vi "Sequence Read.vi"(8 "error in (no error)":errorcluster, 11 "CAP-USB-1 in":refnum<class "CAP-USB-1.lvclass">) -> (0 "error out":errorcluster, 1 "Control Data":T3, 2 "Acquisition Data":T1, 3 "CAP-USB-1 out":refnum<class "CAP-USB-1.lvclass">)   [LabVIEW 2014, in "CAP-USB-1.lvlib" / "CAP-USB-1.lvclass"]
doc: "Realiza la lectura de los valores enviados por el dispositivo en modo sequence"
uses:
  CAP-USB-1.lvclass
  DriverMasterSync/build/DriverMasterSync.lvlibp/APIs/Data Queue/Control Data Cluster.ctl
  DriverMasterSync/build/DriverMasterSync.lvlibp/APIs/Data Queue/Acquisition Data Cluster.ctl
  DriverMasterSync/build/DriverMasterSync.lvlibp/APIs/Data Queue/Acquisition Data 1 Sample Cluster.ctl
  CAP-USB-1.lvclass/CAP-USB-1.ctl
  API/CAP-USB/CAP-USB.lvlib
  DriverMasterSync/build/DriverMasterSync.lvlibp/Modules/HAL/DriverMasterSync/DriverMasterSyncClass/DriverMasterSync.lvclass
  DriverMasterSync/build/DriverMasterSync.lvlibp/APIs/Data Queue/WINFAS 2 Data Queue.lvlib
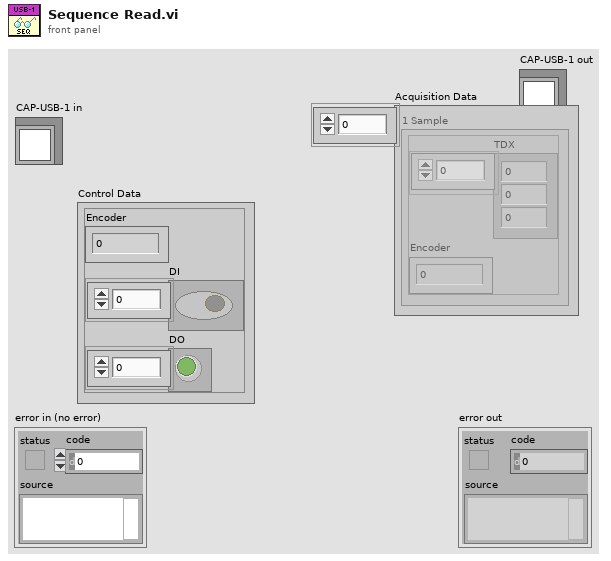
[diagram p1: front panel]
types:
  T1 = typedef "DriverMasterSync.lvlibp/WINFAS 2 Data Queue.lvlib/Acquisition Data Cluster.ctl" = T2[]
  T2 = typedef "DriverMasterSync.lvlibp/WINFAS 2 Data Queue.lvlib/Acquisition Data 1 Sample Cluster.ctl" = cluster{"TDX":sgl[], "Encoder":sgl}
  T3 = typedef "DriverMasterSync.lvlibp/WINFAS 2 Data Queue.lvlib/Control Data Cluster.ctl" = cluster{"Encoder":sgl, "DI":bool[], "DO":bool[]}
  T4 = cluster{"Entradas":bool[], "Salidas":bool[], "Valor Encoder":u16, "Valor Transductores":u16[], "Orden Transd":u32[]}[]
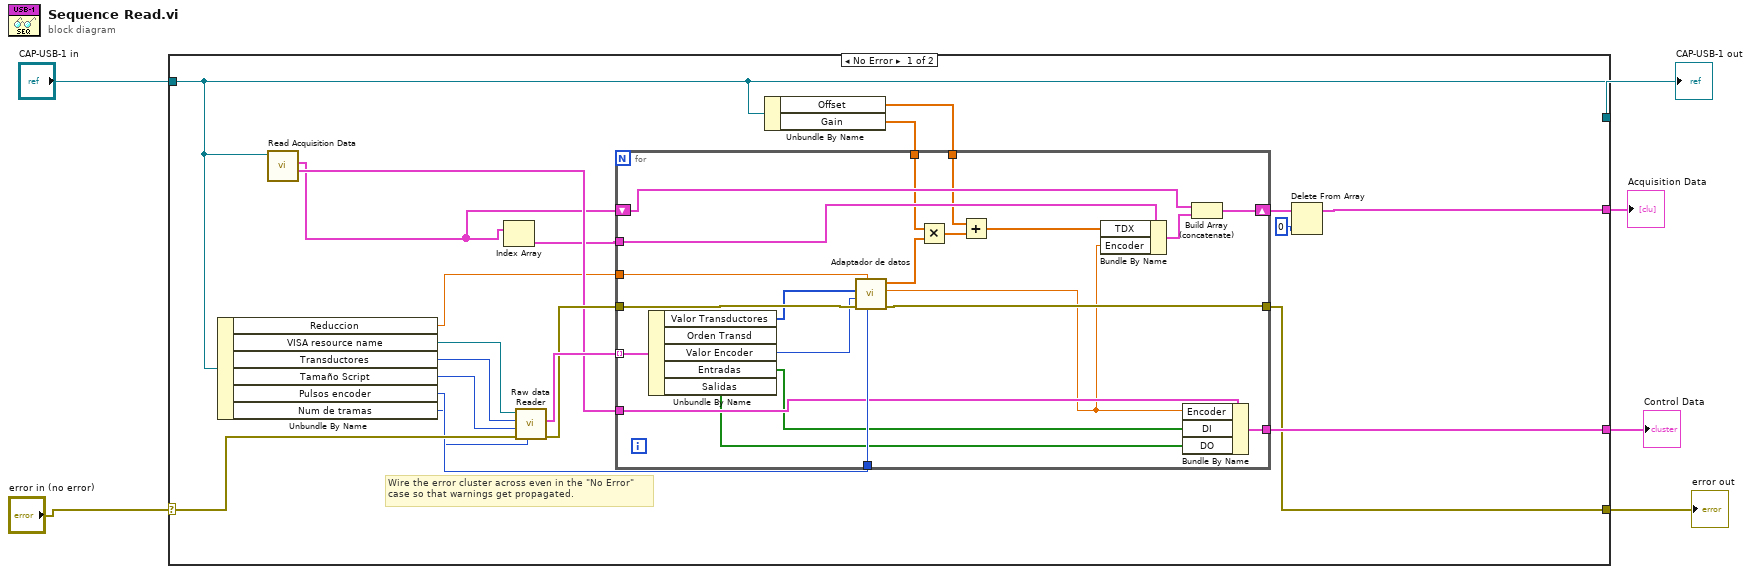
[diagram p0: block diagram]
diagram:
  n1 = case shown="No Error" "error in (no error)" {
    selector: "error in (no error)" -> [w24 w49]
    tunnel: [w11 w49] -> w3
    tunnel: [w10 w48] -> w4
    tunnel: "CAP-USB-1 in" -> [w10 w48]
    tunnel: [w12 _] -> w1
    tunnel: [w17 _] -> w2
    frame No Error {
      # "Wire the error cluster across even in the \"No Error\"\ncase so that warnings get propagated."
      n2 = Unbundle By Name(w10) -> ("Reduccion"=w7:sgl, "VISA resource name"=w22:refnum<visa-resource-name>, "Transductores"=w26:u64, "Tamaño Script"=w25:i32, "Pulsos encoder"=w20:u16, "Num de tramas"=w19:u32)
      n3 = call "Read Acquisition Data.vi"("DriverMasterSync in"=w10) -> ("Control Data"=w18:T3, "Acquisition Data"=w15:T1)  [unwired: 7 in, 2 out]
      n4 = Index Array(array=w15) -> (element=w16:T2)  [unwired: 1 in]
      n5 = call "Raw data Reader.vi"("Num de tramas"=w19, "error in (no error)"=w24, "Tamaño Script"=w25, "TRANSDUCTORES"=w26, "VISA Refnum in"=w22) -> ("error out"=w21:errorcluster, "Raw data"=w23:T4)  [unwired: 2 in, 1 out]
      n6 = Unbundle By Name(w10) -> ("Offset"=w8:sgl[], "Gain"=w9:sgl[])
      n7 = for {
        tunnel: w16 -> [w47]
        tunnel: w23 -> [w46] mode=indexing
        tunnel: w21 -> [w45]
        tunnel: [w44] -> w11
        tunnel: w20 -> [w41]
        tunnel: w18 -> [w40]
        tunnel: [w37] -> w17
        shift-right: [w34] -> w14
        shift-left: w15 -> [w36]
        tunnel: w9 -> [w32]
        tunnel: w8 -> [w30]
        tunnel: w7 -> [w27]
        n8 = Unbundle By Name(w46) -> ("Valor Transductores"=w43:u16[], "Valor Encoder"=w42:u16, "Entradas"=w39:bool[], "Salidas"=w38:bool[])  [unwired: 1 out]
        n9 = call "Adaptador de datos.vi"("Cant. de pulsos"=w41, "Reduccion"=w27, "error in (no error)"=w45, "Encoder"=w42, "Transductores"=w43) -> ("error out"=w44:errorcluster, "Encoder"=w33:sgl, "Transductores"=w29:sgl[])  [unwired: 4 in]
        n10 = Multiply(x=w32, y=w29) -> (x*y=w31:sgl[])
        n11 = Add(x=w30, y=w31) -> (x+y=w28:sgl[])
        n12 = Bundle By Name(cluster=w47, "TDX"=w28, "Encoder"=w33) -> (w35:T2)
        n13 = Bundle By Name(cluster=w40, "Encoder"=w33, "DI"=w39, "DO"=w38) -> (w37:T3)
        n14 = Build Array (concatenate)(w36, w35) -> (w34:T1)
      }
      n15 = Delete From Array(array=w14, index=0) -> (array with subset deleted=w12:T1)  [unwired: 1 in, 1 out]
    }
    frame Error {
    }
  }
  "error out" <- w3
  "CAP-USB-1 out" <- w4
  "Control Data" <- w2
  "Acquisition Data" <- w1
